vi "GetTreeRefnum.vi"(1 "Tree in":refnum<class "Tree.lvclass">) -> (0 "Tree Refnum":refnum<vi>)   [LabVIEW 2021, in "Tree.lvlib" / "Tree.lvclass"]
uses:
  Tree.lvclass
  Tree.lvclass/Tree.ctl
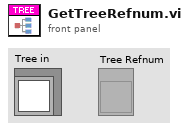
[diagram p1: front panel]
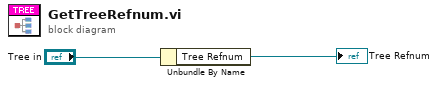
[diagram p0: block diagram]
diagram:
  n1 = Unbundle By Name("Tree in") -> ("Tree Refnum"=→"Tree Refnum":refnum<vi>)
